vi "Add Default Free.vi"(8 "error in (no error)":errorcluster, 10 "ToModBus":bool, 11 "Resistance in":refnum<class "Resistance.lvclass">) -> (0 "error out":errorcluster, 3 "Resistance out":refnum<class "Resistance.lvclass">)   [LabVIEW 2012, in "Measurement Channels.lvlib" / "Resistance.lvclass"]
uses:
  Resistance.lvclass
  Class Channel/Channel.lvclass
  Class Channel/Write Unit_EU.vi
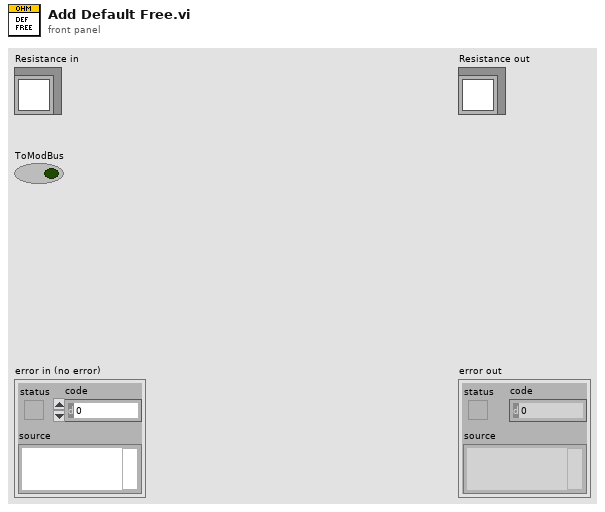
[diagram p1: front panel]
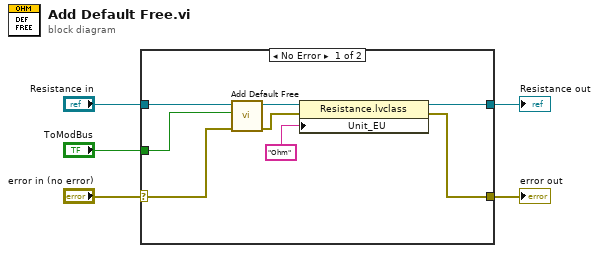
[diagram p0: block diagram]
diagram:
  n1 = case shown="No Error" "error in (no error)" {
    selector: "error in (no error)" -> [w6 w14]
    tunnel: "ToModBus" -> [w13 _]
    tunnel: "Resistance in" -> [w12 w15]
    tunnel: [w8 w15] -> w2
    tunnel: [w7 w14] -> w1
    frame No Error {
      n2 = call-parent "Add Default Free.vi"("error in (no error)"=w6, "ToModBus"=w13, "Channel in"=w12) -> ("error out"=w10:errorcluster, "Channel out"=w11:refnum<class "Resistance.lvclass">)  [unwired: 7 in]
      n3 = property class="Resistance.lvclass"(reference=w11, error in=w10, "Unit_EU"="Ohm") -> (reference out=w8:refnum<class "Resistance.lvclass">, error out=w7:errorcluster)
    }
    frame Error {
    }
  }
  "error out" <- w1
  "Resistance out" <- w2
